vi "Pick A DOF Strategy.vi"(10 "Force Control Parameters":T2) -> (2 "Pick A DOF Strategy":T1)   [LabVIEW 2013]
uses:
  Data Access Objects/Mixed Mode/Force Control Parameters.ctl
  Pick A DOF Strategy Types.ctl
  Data Access Objects/Metadata/DAO Actions.ctl
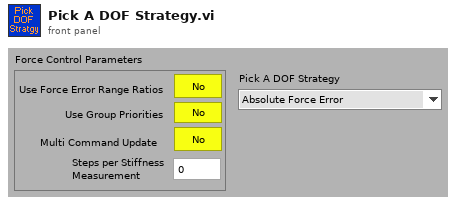
[diagram p1: front panel]
types:
  T1 = typedef "Pick A DOF Strategy Types.ctl" = enum16{"Absolute Force Error", "Normalized Force Error", "Group Priorities Absolute", "Group Priorities Normalized", "Multi DOF Ramp Counting", "Multi DOF Ramp Counting Group", "Multi DOF Stiffness Test"}
  T2 = typedef "Force Control Parameters.ctl" = cluster{"Use Force Error Range Ratios":bool, "Use Group Priorities":bool, "Multi Command Update":bool, "Steps per Stiffness \nMeasurement":i32}
  T3 = typedef "DAO Actions.ctl" = enum16{"Init", "Get", "Set"}
  T4 = typedef "Mixed Mode Multidof Status.ctl" = cluster{"Mixed Mode Multidof State":T5, "Multi DOF Ramp Count":i32, "Stiffness Tested":T6[][]}
  T5 = typedef "Mixed Mode Multidof State.ctl" = enum16{"Multidof", "Stiffness Test", "Start Iterative Stage"}
  T6 = typedef "Yes No Button.ctl" = bool
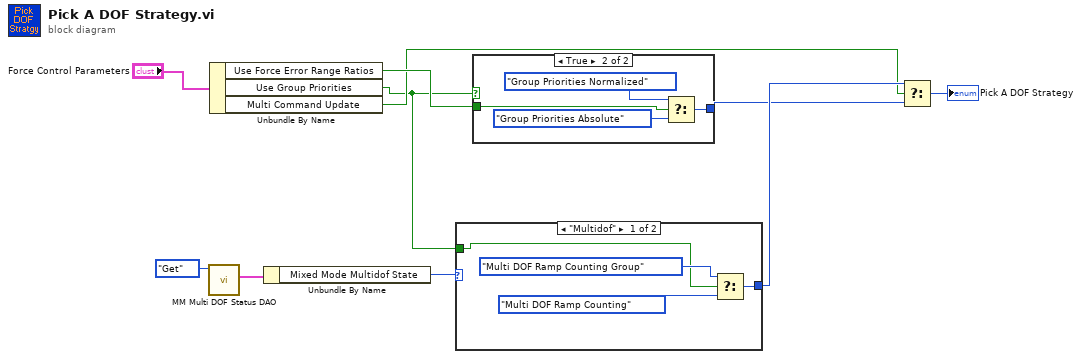
[diagram p0: block diagram]
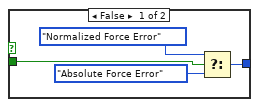
[diagram p2: hidden frame]
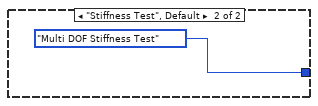
[diagram p3: hidden frame]
diagram:
  n1 = call "MM Multi DOF Status DAO.vi"("Actions"=DAO_Actions."Get") -> ("Mixed Mode Multidof Status Out"=w8:T4)  [unwired: 9 in, 1 out]
  n2 = Unbundle By Name("Force Control Parameters") -> ("Use Force Error Range Ratios"=w3:bool, "Use Group Priorities"=w1:bool, "Multi Command Update"=w2:bool)
  n3 = Unbundle By Name(w8) -> ("Mixed Mode Multidof State"=w7:T5)
  n4 = case shown="\"Multidof\"" w7 {
    tunnel: [w13 Pick_A_DOF_Strategy_Types."Multi DOF Stiffness Test" ("Pick A DOF Strategy")] -> w6
    tunnel: w1 -> [w11 _]
    frame "Multidof" {
      n5 = Select(t=Pick_A_DOF_Strategy_Types."Multi DOF Ramp Counting Group", s=w11, f=Pick_A_DOF_Strategy_Types."Multi DOF Ramp Counting" ("Pick A DOF Strategy")) -> (s? t:f=w13:T1)
    }
    frame "Stiffness Test", Default {
    }
  }
  n6 = case shown="True" w1 {
    tunnel: [w17 w21] -> w4
    tunnel: w3 -> [w16 w20]
    frame False {
      n7 = Select(t=Pick_A_DOF_Strategy_Types."Normalized Force Error", s=w16, f=Pick_A_DOF_Strategy_Types."Absolute Force Error" ("Pick A DOF Strategy")) -> (s? t:f=w17:T1)
    }
    frame True {
      n8 = Select(t=Pick_A_DOF_Strategy_Types."Group Priorities Normalized", s=w20, f=Pick_A_DOF_Strategy_Types."Group Priorities Absolute" ("Pick A DOF Strategy")) -> (s? t:f=w21:T1)
    }
  }
  n9 = Select(t=w6, s=w2, f=w4) -> (s? t:f=→"Pick A DOF Strategy":T1)
